vi "kDSA01.vi"(8 "DSA Control Variables":T1={"High Freq"=200.0, "Sample Time"=0.001, "Low Freq"=10.0, "Num Data Points"=10, "Num Periods"=10, "Settling Time"=0.1}, 11 "Sensor Reading":dbl) -> (0 "Imag":dbl[](array[numeric]), 1 "Re":dbl[](array[numeric]), 2 "Frequencies":dbl[](array[numeric]), 3 "excitation signal":dbl)   [LabVIEW 2011, in "kevLib2011.lvlib"]
uses:
  kevLib2011.lvlib
  DSACntVariables.ctl
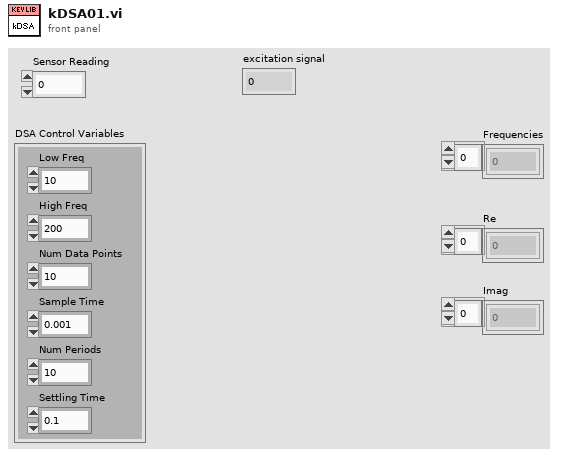
[diagram p1: front panel]
types:
  T1 = typedef "kevLib2011.lvlib/DSACntVariables.ctl" = cluster{"High Freq":dbl, "Sample Time":dbl, "Low Freq":dbl, "Num Data Points":i32, "Num Periods":i32, "Settling Time":dbl}
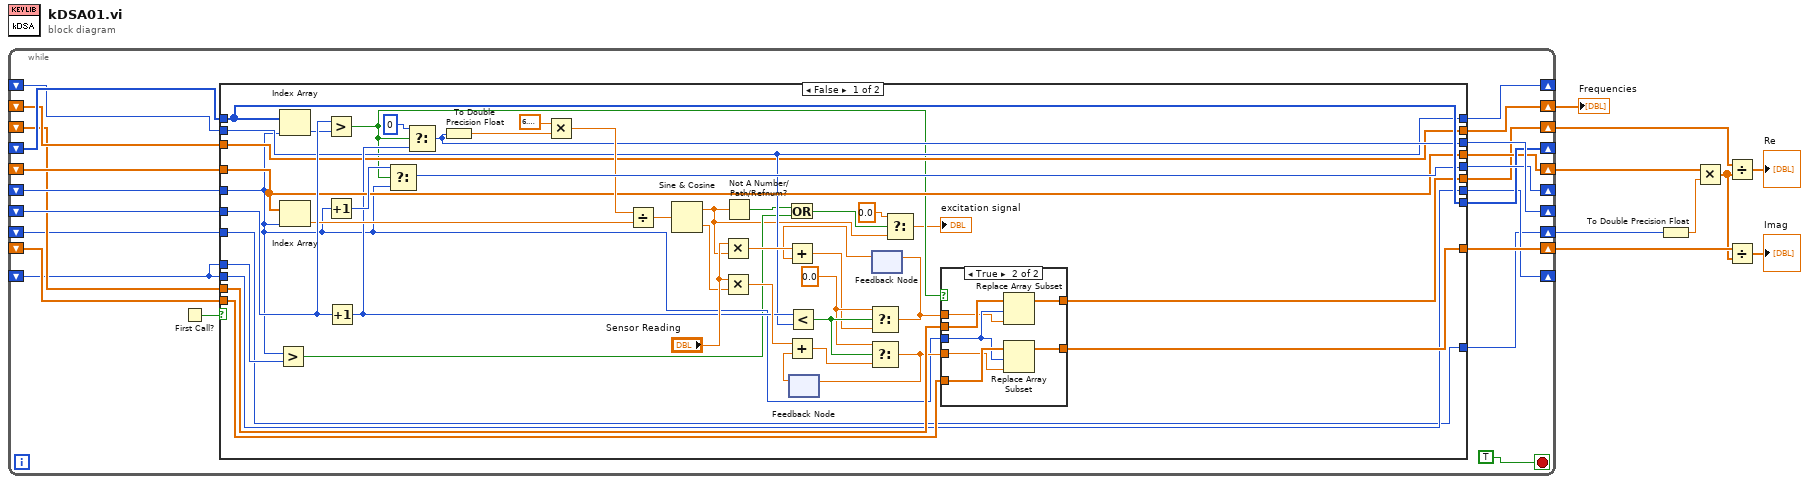
[diagram p0: block diagram]
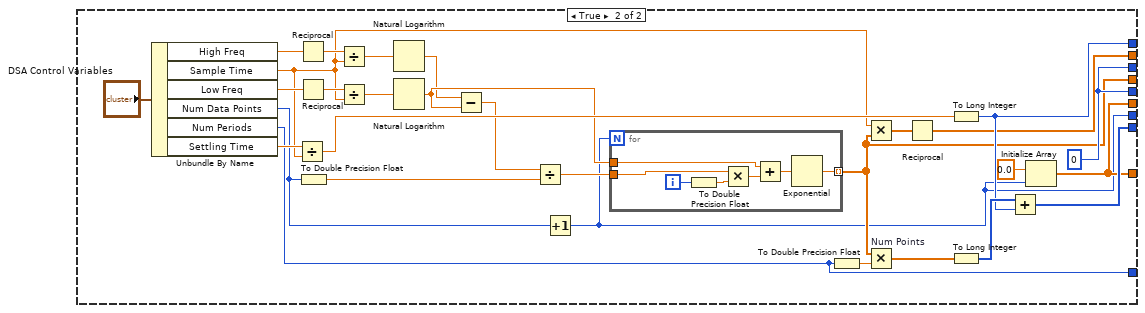
[diagram p3: hidden frame]
diagram:
  n1 = while {
    shift-right: [w29] -> _
    shift-left: _ -> [w28]
    shift-right: [w27] -> _
    shift-left: _ -> [w26]
    shift-right: [w25] -> _
    shift-left: _ -> [w24]
    shift-right: [w23] -> w2
    shift-left: _ -> [w22]
    shift-right: [w21] -> _
    shift-left: _ -> [w20]
    shift-right: [w17] -> w9
    shift-left: _ -> [w16]
    shift-right: [w19] -> w5
    shift-left: _ -> [w15]
    shift-right: [w18] -> w7
    shift-left: _ -> [w14]
    shift-right: [w13] -> _
    shift-left: _ -> [w12]
    shift-right: [w11] -> w3
    shift-left: _ -> [w10]
    stop <- TRUE stop-if-true
    n2 = First Call?() -> (First Call?: T/F=w30:bool)
    n3 = case shown="False" w30 {
      tunnel: [w64 w96] -> w29
      tunnel: w28 -> [w73 _]
      tunnel: [w69 w96] -> w27
      tunnel: w26 -> [w40 _]
      tunnel: [w72 w94] -> w25
      tunnel: w24 -> [w72 _]
      tunnel: [w63 w88] -> w23
      tunnel: w22 -> [w63 _]
      tunnel: [w56 w92] -> w21
      tunnel: w20 -> [w56 _]
      tunnel: [w44 w86] -> w19
      tunnel: [w43 w86] -> w18
      tunnel: [w49 w89] -> w17
      tunnel: w16 -> [w49 _]
      tunnel: w15 -> [w48 _]
      tunnel: w14 -> [w47 _]
      tunnel: [w41 w85] -> w13
      tunnel: w12 -> [w41 _]
      tunnel: w12 -> [w39 _]
      tunnel: [w32 w84] -> w11
      tunnel: w10 -> [w32 _]
      frame False {
        w54 = 0.0 ("t")
        n4 = Greater?(x=w40, y=w39) -> (0:w35:bool)
        n5 = Index Array(array=w72, index=w40) -> (element=w71:i32)
        n6 = Index Array(array=w63, index=w40) -> (element=w62:dbl)
        n7 = Greater?(x=w73, y=w71) -> (0:w42:bool)
        n8 = Increment(x=w40) -> (x+1=w70:i32)
        n9 = Increment(x=w73) -> (x+1=w57:i32)
        n10 = Select(t=w70, s=w42, f=w40) -> (s? t:f=w69:i32)
        n11 = Select(t=0, s=w42, f=w57) -> (s? t:f=w64:i32)
        n12 = To Double Precision Float(number=w64) -> (double precision float=w65:dbl)
        n13 = Multiply(x=6.283185307179586, y=w65) -> (x*y=w67:dbl)
        n14 = Divide(x=w67, y=w62) -> (x/y=w68:dbl)
        n15 = Sine & Cosine(0:w68) -> (1:w33:dbl, 2:w60:dbl)
        n16 = Multiply(x="Sensor Reading", y=w33) -> (x*y=w59:dbl)
        n17 = Multiply(x="Sensor Reading", y=w60) -> (x*y=w58:dbl)
        n18 = Not A Number/Path/Refnum?(number/path/refnum=w33) -> (NaN/Path/Refnum?=w36:bool)
        n19 = Or(x=w36, y=w35) -> (x .or. y?=w34:bool)
        n20 = Less?(x=w57, y=w56) -> (x < y?=w55:bool)
        n21 = feedback #1() -> (w51:dbl)  [unwired: 1 in]
        n22 = Add(x=w58, y=w51) -> (x+y=w50:dbl)
        n23 = Select(t=w54, s=w55, f=w50) -> (s? t:f=w45:dbl)
        n24 = feedback-in #1(w45) -> ()
        n25 = feedback #2() -> (w53:dbl)  [unwired: 1 in]
        n26 = Add(x=w59, y=w53) -> (x+y=w52:dbl)
        n27 = Select(t=w54, s=w55, f=w52) -> (s? t:f=w46:dbl)
        n28 = feedback-in #2(w46) -> ()
        n29 = Select(t=0.0, s=w34, f=w33) -> (s? t:f=→"excitation signal":dbl)
        n30 = case shown="True" w42 {
          tunnel: w48 -> [w76 w83]
          tunnel: w47 -> [w75 w82]
          tunnel: w40 -> [_ w81]
          tunnel: w46 -> [_ w80]
          tunnel: w45 -> [_ w79]
          tunnel: [w76 w78] -> w44
          tunnel: [w75 w77] -> w43
          frame False {
          }
          frame True {
            n31 = Replace Array Subset(array=w83, new element=w80, index=w81) -> (w78:dbl[])
            n32 = Replace Array Subset(array=w82, new element=w79, index=w81) -> (w77:dbl[])
          }
        }
      }
      frame True {
        w96 = 0 ("32bit integer")
        n33 = Unbundle By Name("DSA Control Variables") -> ("High Freq"=w109:dbl, "Sample Time"=w90:dbl, "Low Freq"=w110:dbl, "Num Data Points"=w111:i32, "Num Periods"=w84:i32, "Settling Time"=w112:dbl)
        n34 = Divide(x=w112, y=w90) -> (x/y=w104:dbl)
        n35 = Reciprocal(x=w109) -> (1/x=w106:dbl)
        n36 = Reciprocal(x=w110) -> (1/x=w105:dbl)
        n37 = To Double Precision Float(number=w111) -> (double precision float=w99:dbl)
        n38 = Divide(x=w106, y=w90) -> (x/y=w103:dbl)
        n39 = Divide(x=w105, y=w90) -> (x/y=w102:dbl)
        n40 = Natural Logarithm(1:w103) -> (0:w97:dbl)
        n41 = Natural Logarithm(1:w102) -> (0:w101:dbl)
        n42 = Subtract(x=w97, y=w101) -> (x-y=w98:dbl)
        n43 = Divide(x=w98, y=w99) -> (x/y=w100:dbl)
        n44 = Increment(x=w111) -> (x+1=w85:i32)
        n45 = for {
          N: w85 -> [_]
          tunnel: w100 -> [w117]
          tunnel: w101 -> [w116]
          tunnel: [w113] -> w88 mode=indexing
          i -> [w119]
          n46 = To Double Precision Float(number=w119) -> (double precision float=w118:dbl)
          n47 = Multiply(x=w117, y=w118) -> (x*y=w115:dbl)
          n48 = Add(x=w116, y=w115) -> (x+y=w114:dbl)
          n49 = Exponential(1:w114) -> (0:w113:dbl)
        }
        n50 = To Double Precision Float(number=w84) -> (double precision float=w107:dbl)
        n51 = Multiply(x=w90, y=w88) -> (x*y=w91:dbl[])
        n52 = Multiply "Num Points"(x=w88, y=w107) -> (x*y=w93:dbl[])
        n53 = Reciprocal(x=w91) -> (1/x=w89:dbl[])
        n54 = To Long Integer(number=w104) -> (32bit integer=w92:i32)
        n55 = To Long Integer(number=w93) -> (32bit integer=w95:i32[])
        n56 = Add(x=w95, y=w92) -> (x+y=w94:i32[])
        n57 = Initialize Array(0.0 ("element"), w85) -> (w86:dbl[])
      }
    }
  }
  "Frequencies" <- w9
  n58 = To Double Precision Float(number=w3) -> (double precision float=w4:dbl)
  n59 = Multiply(x=w2, y=w4) -> (x*y=w1:dbl[])
  n60 = Divide(x=w5, y=w1) -> (x/y=→"Re":dbl[])
  n61 = Divide(x=w7, y=w1) -> (x/y=→"Imag":dbl[])
